vi "LDT Parse XML AOS.vi"(11 "AOS Status XML":string) -> (2 "total focus offset (um)":dbl, 3 "Settled":bool)   [LabVIEW 2022 SP3, in "LDT Telescope.lvclass"]
uses:
  LDT Telescope.lvclass
panel:
  out "Array":bool[](array[boolean])
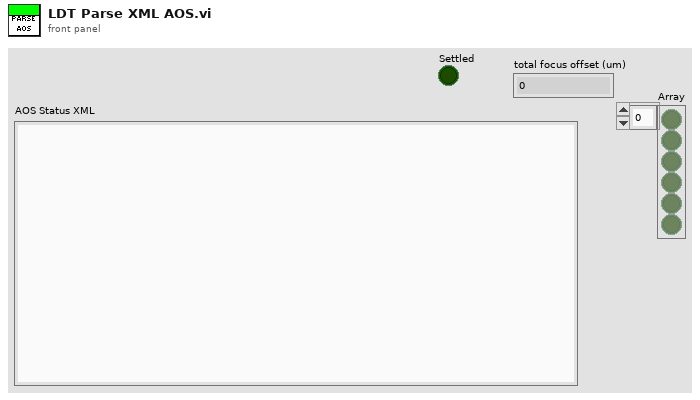
[diagram p1: front panel]
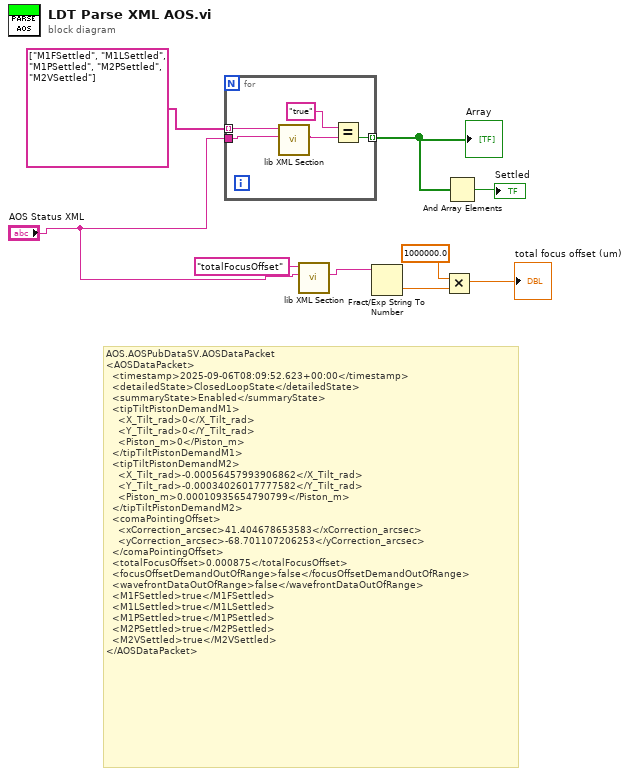
[diagram p0: block diagram]
diagram:
  # "AOS.AOSPubDataSV.AOSDataPacket\n<AOSDataPacket>\n  <timestamp>2025-09-06T08:09:52.623+00:00</timestamp>\n  <detailedState>ClosedLoopState</detailedState>\n  <summaryState>Enabled</summaryState>\n  <tipTiltPistonDemandM1>\n    <X_Tilt_rad>0</X_Tilt_rad>\n    <Y_Tilt_rad>0</Y_Tilt_rad>\n    <Piston_m>0</Piston_m>\n  </tipTiltPistonDemandM1>\n  <tipTiltPistonDemandM2>\n    <X_Tilt_rad>-0.00056457993906862</X_Tilt_rad>\n    <Y_Tilt_rad>-0.00034026017777582</Y_Tilt_rad>\n    <Piston_m>0.00010935654790799</Piston_m>\n  </tipTiltPistonDemandM2>\n  <comaPointingOffset>\n    <xCorrection_arcsec>41.404678653583</xCorrection_arcsec>\n    <yCorrection_arcsec>-68.701107206253</yCorrection_arcsec>\n  </comaPointingOffset>\n  <totalFocusOffset>0.000875</totalFocusOffset>\n  <focusOffsetDemandOutOfRange>false</focusOffsetDemandOutOfRange>\n  <wavefrontDataOutOfRange>false</wavefrontDataOutOfRange>\n  <M1FSettled>true</M1FSettled>\n  <M1LSettled>true</M1LSettled>\n  <M1PSettled>true</M1PSettled>\n  <M2PSettled>true</M2PSettled>\n  <M2VSettled>true</M2VSettled>\n</AOSDataPacket>"
  n1 = for {
    tunnel: string[] ["M1FSettled", "M1LSettled", "M1PSettled", "M2PSettled", "M2VSettled"] -> [w14] mode=indexing
    tunnel: "AOS Status XML" -> [w13]
    tunnel: [w11] -> w8 mode=indexing
    n2 = call "lib XML Section.vi"("XML String"=w13, "XML Topic"=w14) -> ("XML Topic Body"=w12:string)  [unwired: 6 in, 3 out]
    n3 = Equal?(x="true", y=w12) -> (x = y?=w11:bool)
  }
  "Array" <- w8
  n4 = call "lib XML Section.vi"("XML String"="AOS Status XML", "XML Topic"="totalFocusOffset") -> ("XML Topic Body"=w4:string)  [unwired: 6 in, 3 out]
  n5 = Fract/Exp String To Number(string=w4) -> (number=w3:dbl)  [unwired: 3 in, 1 out]
  n6 = Multiply(x=1000000.0, y=w3) -> (x*y=→"total focus offset (um)":dbl)
  n7 = And Array Elements(Boolean array=w8) -> (logical AND=→"Settled":bool)
